vi "Pre Launch Init.vi"(11 "Heater in":refnum<class "Heater.lvclass">) -> (0 "error out":errorcluster, 3 "Heater out":refnum<class "Heater.lvclass">)   [LabVIEW 2015, in "cRIO-Carbondioxide.lvlib" / "CO2-Actor.lvlib" / "Heater.lvclass"]
doc: "(<B>Filename</B>: Actor Framework.lvlib:Actor.lvclass:Pre Launch Init.vi)\n\nDefines behavior that occurs after the Launch Actor method is invoked but before the actor's Actor Core method begins running.\n\nThe Pre Launch Init method is guaranteed to finish before the Launch Actor method returns to its caller and before the actor itself receives any messages. Any references that the Pre Launch Init method obtains are guaranteed to have the same lifetime as the actor itself. Any errors that the Pre Launch Init method returns will abort the launch.\n\nBy default, this method does nothing. A descendant class may override it to define behavior."
uses:
  Heater.lvclass
  CO2 Actor/CO2 Actor.lvclass
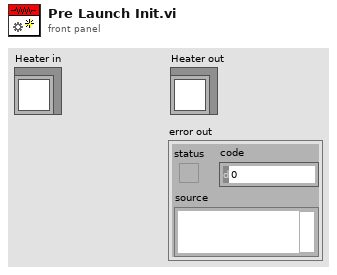
[diagram p1: front panel]
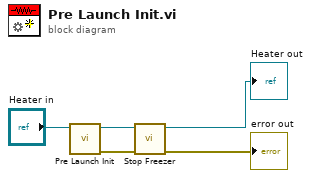
[diagram p0: block diagram]
diagram:
  n1 = call-parent "Pre Launch Init.vi"("CO2 Actor in"="Heater in") -> ("error out"=w4:errorcluster, "CO2 Actor out"=w2:refnum<class "Heater.lvclass">)  [unwired: 9 in]
  n2 = call "Stop Freezer.vi"("error in (no error)"=w4, "Heater in"=w2) -> ("error out"=→"error out":errorcluster, "Heater out"=→"Heater out":refnum<class "Heater.lvclass">)  [unwired: 8 in]
